vi "Create Platform Endpoint.vi"(6 "User Data":string, 7 "Region":T1, 8 "error in (no error)":errorcluster, 10 "Platform Application":refnum<class "Platform Application.lvclass">, 11 "AWS Credentials":T2) -> (0 "error out":errorcluster, 3 "Endpoint out":refnum<class "Endpoint.lvclass">)   [LabVIEW 2015, in "NI_AWS_SNS.lvlib" / "Endpoint.lvclass"]
uses:
  Endpoint.lvclass
  Core/HTTP Request/AWS Credentials.ctl
  Core/HTTP Request/Region.ctl
  Platform Application/Platform Application.lvclass
  Core/HTTP Request/Request Options.ctl
  Core/HTTP Request/Name Value Pair.ctl
  Core/HTTP Request/Region handling.ctl
  Core/HTTP Request/URL formatting.ctl
  Core/ARN/ARN.lvclass/ARN.ctl
  Core/ARN/Read ARN.vi
  Core/HTTP Request/HTTP Request.lvclass
  Core/ARN/ARN.lvclass
panel:
  in  "Token":string
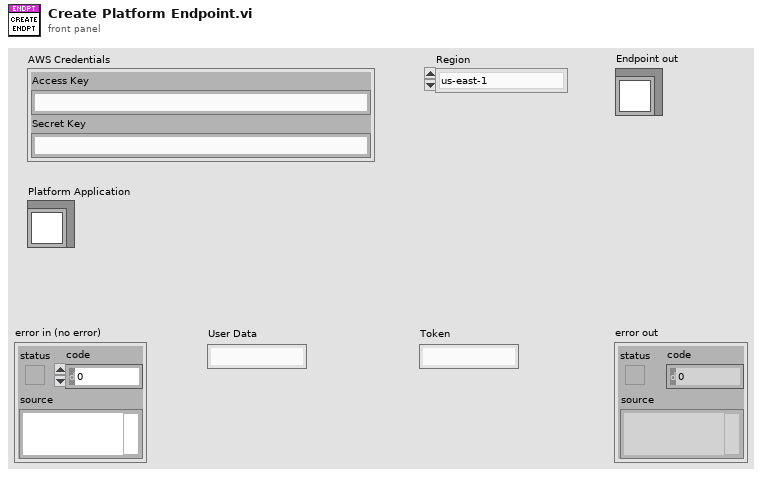
[diagram p1: front panel]
types:
  T1 = typedef "NI_AWS_Core.lvlib/HTTP Request.lvclass/Region.ctl" = enum16{"us-east-1", "us-east-2", "us-west-1", "us-west-2", "ap-northeast-1", "ap-northeast-2", "ap-southeast-1", "ap-southeast-2", "ca-central-1", "eu-central-1", "eu-west-1", "eu-west-2", "sa-east-1"}
  T2 = typedef "NI_AWS_Core.lvlib/HTTP Request.lvclass/AWS Credentials.ctl" = cluster{"Access Key":string, "Secret Key":string}
  T3 = typedef "NI_AWS_Core.lvlib/HTTP Request.lvclass/Name Value Pair.ctl" = cluster{"name":string, "value":string}
  T4 = typedef "NI_AWS_Core.lvlib/HTTP Request.lvclass/Request Options.ctl" = cluster{"request headers":T3[], "request parameters":T3[], "request body":string, "region handling":T5, "URL formatting":T6}
  T5 = typedef "NI_AWS_Core.lvlib/HTTP Request.lvclass/Region handling.ctl" = enum16{"use region everywhere", "use region (authentication only)", "use region (URL only)", "ignore region everwhere"}
  T6 = typedef "NI_AWS_Core.lvlib/HTTP Request.lvclass/URL formatting.ctl" = enum16{"region-", "region."}
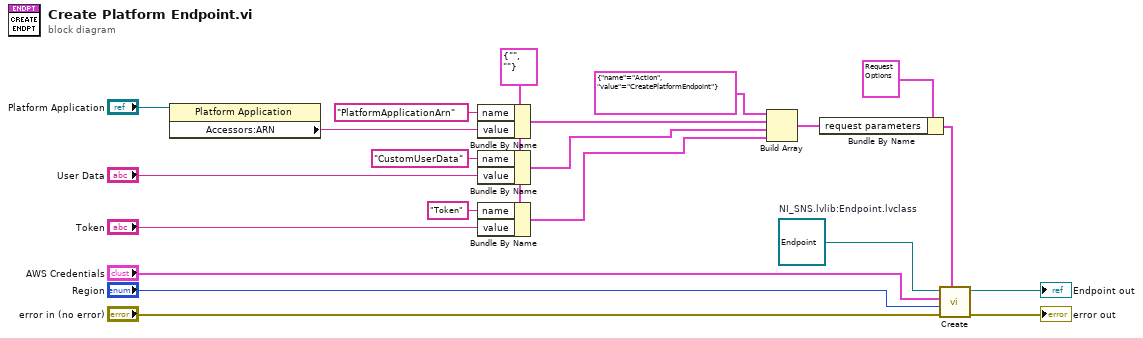
[diagram p0: block diagram]
diagram:
  w9 = refnum<class "Endpoint.lvclass"> refnum  # NI_SNS.lvlib:Endpoint.lvclass
  w12 = T3 {"name"="", "value"=""} ("element")
  n1 = property class="Platform Application"(reference="Platform Application") -> ("Accessors:ARN"=w15:string)  [unwired: 1 in, 2 out]
  n2 = Bundle By Name(cluster=w12, "name"="PlatformApplicationArn", "value"=w15) -> (w18:T3)
  n3 = Bundle By Name(cluster=w12, "name"="CustomUserData", "value"="User Data") -> (w11:T3)
  n4 = Bundle By Name(cluster=w12, "name"="Token", "value"="Token") -> (w10:T3)
  n5 = Build Array(T3 {"name"="Action", "value"="CreatePlatformEndpoint"} ("Name Value Pair"), w18, w11, w10) -> (w17:T3[])
  n6 = Bundle By Name(cluster=T4 {"request headers"=[], "request parameters"=[{"name"="Action", "value"="ListQueues"}], "request body"="", "region handling"=enum."use region everywhere", "URL formatting"=enum."region."} ("Request Options"), "request parameters"=w17) -> (w20:T4)
  n7 = call "Create.vi"("Request Options"=w20, "error in (no error)"="error in (no error)", "Region"="Region", "AWS Credentials"="AWS Credentials", "ARN in"=w9) -> ("error out"=→"error out":errorcluster, "ARN out"=→"Endpoint out":refnum<class "Endpoint.lvclass">)  [unwired: 5 in]
